vi "GetEvtSignal.vi"(8 "error in (no error)":errorcluster, 11 "EventFromCSVPlugin in":refnum<class "EventFromCSVPlugin.lvclass">) -> (0 "error out":errorcluster, 3 "EventFromCSVPlugin out":refnum<class "EventFromCSVPlugin.lvclass">)   [LabVIEW 2014, in "EventPlugins.lvlib" / "EventFromCSVPlugin.lvclass"]
uses:
  EventFromCSVPlugin.lvclass
  EventPluginBaseClass/EventPluginBaseClass.lvclass
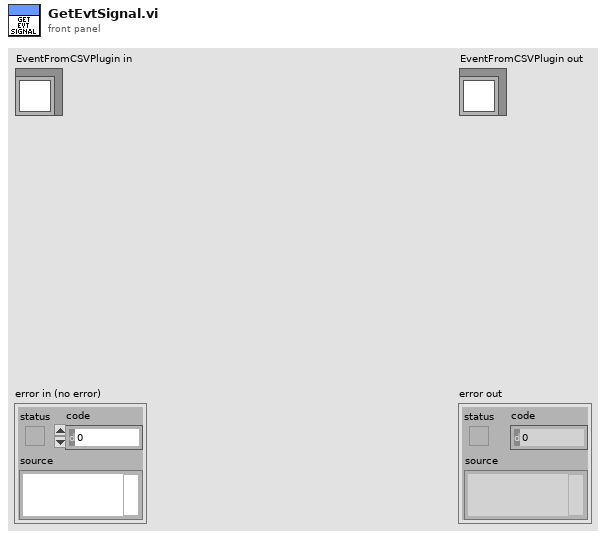
[diagram p1: front panel]
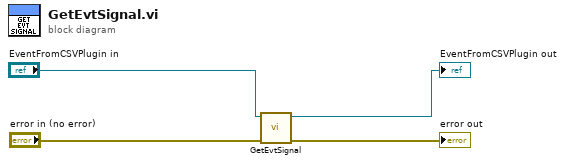
[diagram p0: block diagram]
diagram:
  n1 = call-parent "GetEvtSignal.vi"("error in (no error)"="error in (no error)", "EventPluginBaseClass in"="EventFromCSVPlugin in") -> ("error out"=→"error out":errorcluster, "EventPluginBaseClass out"=→"EventFromCSVPlugin out":refnum<class "EventFromCSVPlugin.lvclass">)  [unwired: 8 in]
